vi "AlliGator Decay Fit Parameter Map Size Dialog.vi"(8 "error in (no error)":errorcluster, 9 "Y Resolution":i32, 10 "X Resolution":i32, 11 "Message":string="No dataset is currently loaded.\nEither load the dataset corresponding to the Decay Fit Parameter Map first, or provide the original dataset's X and Y resolution:") -> (0 "error out":errorcluster, 1 "Y Resolution":i32, 2 "X Resolution":i32, 4 "OK":bool)   [LabVIEW 2021, in "AlliGator Parameter Map.lvlib"]
doc: "Displays a standard dialog box that prompts users to enter information, such as a user name and password.\n--------------------\n\nThis Express VI is configured as follows:\n\nMessage to Display to the User:No dataset is currently loaded.\nEither load the dataset corresponding to the Decay Fit Parameter Map first, or provide the original dataset's X and Y resolution.\nThe inputs are: \nNumber: X Resolution\nNumber: Y Resolution"
uses:
  Parameter Map/AlliGator Parameter Map.lvlib
panel:
  out "String":string="No dataset is currently loaded.\nEither load the dataset corresponding to the Decay Fit Parameter Map first, or provide the original dataset's X and Y resolution."
  in  "Enable":bool=TRUE
  in  "Cancel":bool
  in  "OK`":bool caption="OK2"
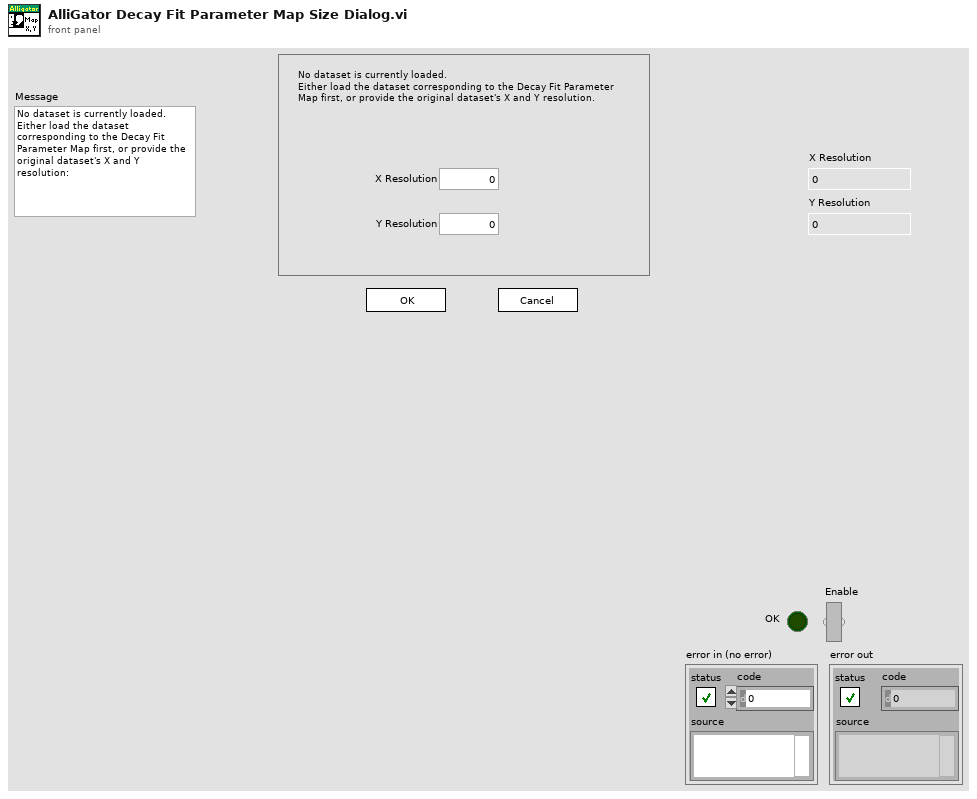
[diagram p1: front panel]
types:
  T1 = cluster{"Input Name":string, "Input Data Type":i32}[]
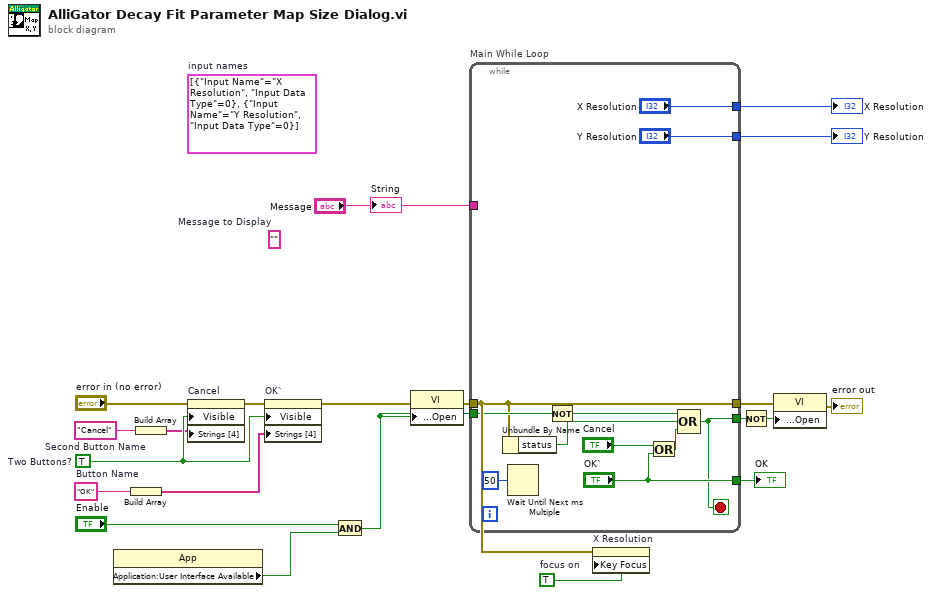
[diagram p0: block diagram]
diagram:
  w5 = TRUE  # focus on
  (unwired) T1 [{"Input Name"="X Resolution", "Input Data Type"=0}, {"Input Name"="Y Resolution", "Input Data Type"=0}]  # input names
  w15 = "Cancel"  # Second Button Name
  w13 = "OK"  # Button Name
  (unwired) ""  # Message to Display
  w21 = TRUE  # Two Buttons?
  n1 = property class="App"() -> ("Application:User Interface Available"=w6:bool)  [unwired: 2 in, 2 out]
  n2 = Build Array(w13) -> (w14:string[])
  n3 = Build Array(w15) -> (w16:string[])
  n4 = property on="Cancel" class="Bool"(error in="error in (no error)", "Visible"=w21, "Strings [4]"=w16) -> (error out=w19:errorcluster)  [unwired: 1 in, 1 out]
  n5 = property on="OK`" class="Bool"(error in=w19, "Visible"=w21, "Strings [4]"=w14) -> (error out=w2:errorcluster)  [unwired: 1 in, 1 out]
  n6 = And(x="Enable", y=w6) -> (x .and. y?=w7:bool)
  n7 = property class="VI"(error in=w2, "Front Panel Window:Open"=w7) -> (error out=w12:errorcluster)  [unwired: 1 in, 1 out]
  n8 = while "Main While Loop" {
    tunnel: ["OK`"] -> w20
    tunnel: w7 -> [w29]
    tunnel: [w27] -> w17
    tunnel: w12 -> [w26]
    tunnel: [w26] -> w10
    tunnel: ["X Resolution"] -> w4
    tunnel: ["Y Resolution"] -> w3
    tunnel: "Message" -> [_]
    stop <- w27 stop-if-true
    n9 = Unbundle By Name(w26) -> ("status"=w24:bool)
    n10 = Wait Until Next ms Multiple(millisecond multiple=u32 50) -> ()  [unwired: 1 out]
    n11 = Not(x=w29) -> (.not. x?=w28:bool)
    n12 = Or(x="Cancel", y="OK`") -> (x .or. y?=w25:bool)
    n13 = Compound Arithmetic op=OR(w28, w24, w25) -> (w27:bool)
  }
  "OK" <- w20
  "X Resolution" <- w4
  "Y Resolution" <- w3
  n14 = property on="X Resolution" class="DigNum (strict)"(error in=w12, "Key Focus"=w5) -> ()  [unwired: 1 in, 2 out]
  n15 = Not(x=w17) -> (.not. x?=w18:bool)
  n16 = property class="VI"(error in=w10, "Front Panel Window:Open"=w18) -> (error out=→"error out":errorcluster)  [unwired: 1 in, 1 out]
  "String" <- "Message"
